vi "Execute actionbackup.vi"(8 "error in (no error)":errorcluster, 10 "Action":string, 11 "Class path":path) -> (0 "error out":errorcluster)   [LabVIEW 2021]
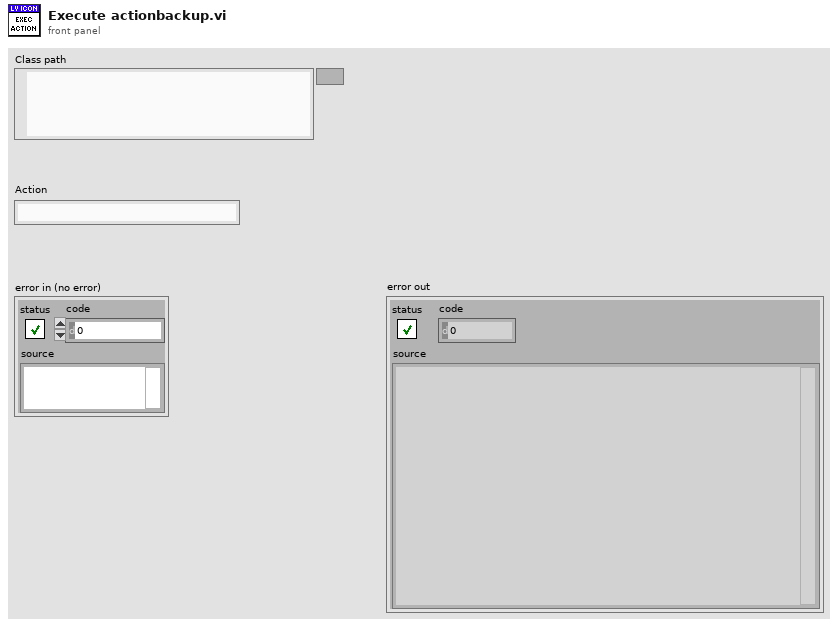
[diagram p1: front panel]
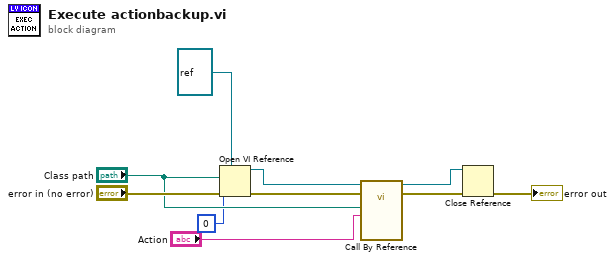
[diagram p0: block diagram]
diagram:
  n1 = Open VI Reference(type specifier VI Refnum (for type only)=refnum<vi> refnum, vi path="Class path", options=0, error in (no error)="error in (no error)") -> (vi reference=w8:refnum<vi>, error out=w9:errorcluster)  [unwired: 2 in]
  n2 = call-by-ref "?"(reference=w8, error in=w9, "Action"="Action", "Class"="Class path") -> (reference out=w1:refnum<vi>, error out=w3:errorcluster)  [unwired: 9 in, 1 out]
  n3 = Close Reference(reference=w1, error in (no error)=w3) -> (error out=→"error out":errorcluster)
